vi "Main.vi"(8 "error in":errorcluster, 11 "CPU Percent in":refnum<class "Place Temperature.lvclass">) -> (0 "error out":errorcluster, 3 "CPU Percent out":refnum<class "Place Temperature.lvclass">)   [LabVIEW 2024, in "Place Temperature.lvclass"]
doc: "The <b>Queued Message Handler</b> of the Worker that owns this VI."
uses:
  Place Temperature.lvclass
  C:/Program Files (x86)/National Instruments/LabVIEW 2024/vi.lib/addons/_Workers/Library/Classes/Worker/Worker.lvclass
  rwr_Get Place Temperature Reply.ctl
  rqp_Set Place.ctl
  Place Temperature.lvclass/Place Temperature.ctl
  Controller/Controller.lvclass
  <vilib>/Python/Open Venv Python Session.vi
  <vilib>/addons/_Workers/Library/Classes/Worker/Worker.lvclass
  <vilib>/addons/_Workers/Library/Classes/Message Queue/Message Queue.lvclass
  Initialization Data.ctl
panel:
  out "Reply Data out":T1
  in  "Places":string(combo)="Baden, CH"
  in  "bGet Temperature":bool
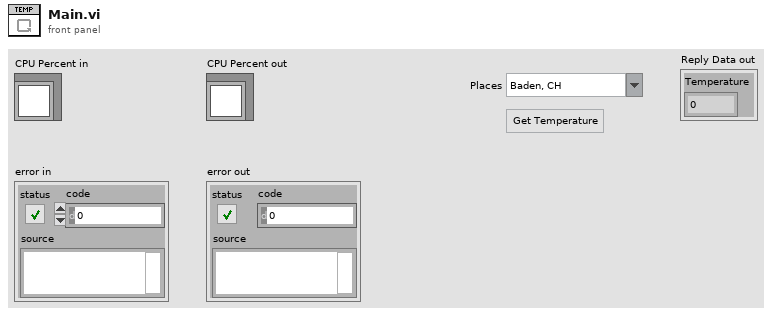
[diagram p1: front panel]
types:
  T1 = typedef "Place Temperature.lvclass/rwr_Get Place Temperature Reply.ctl" = cluster{"Temperature":dbl}
  T2 = typedef "Place Temperature.lvclass/Initialization Data.ctl" = cluster{"String":string, "Show Frontpanel":bool}
  T3 = enum32{"Invalid", "Standard", "Closed", "Hidden", "Minimized", "Maximized"}
  T4 = typedef "Place Temperature.lvclass/rqp_Set Place.ctl" = cluster{"Place":string}
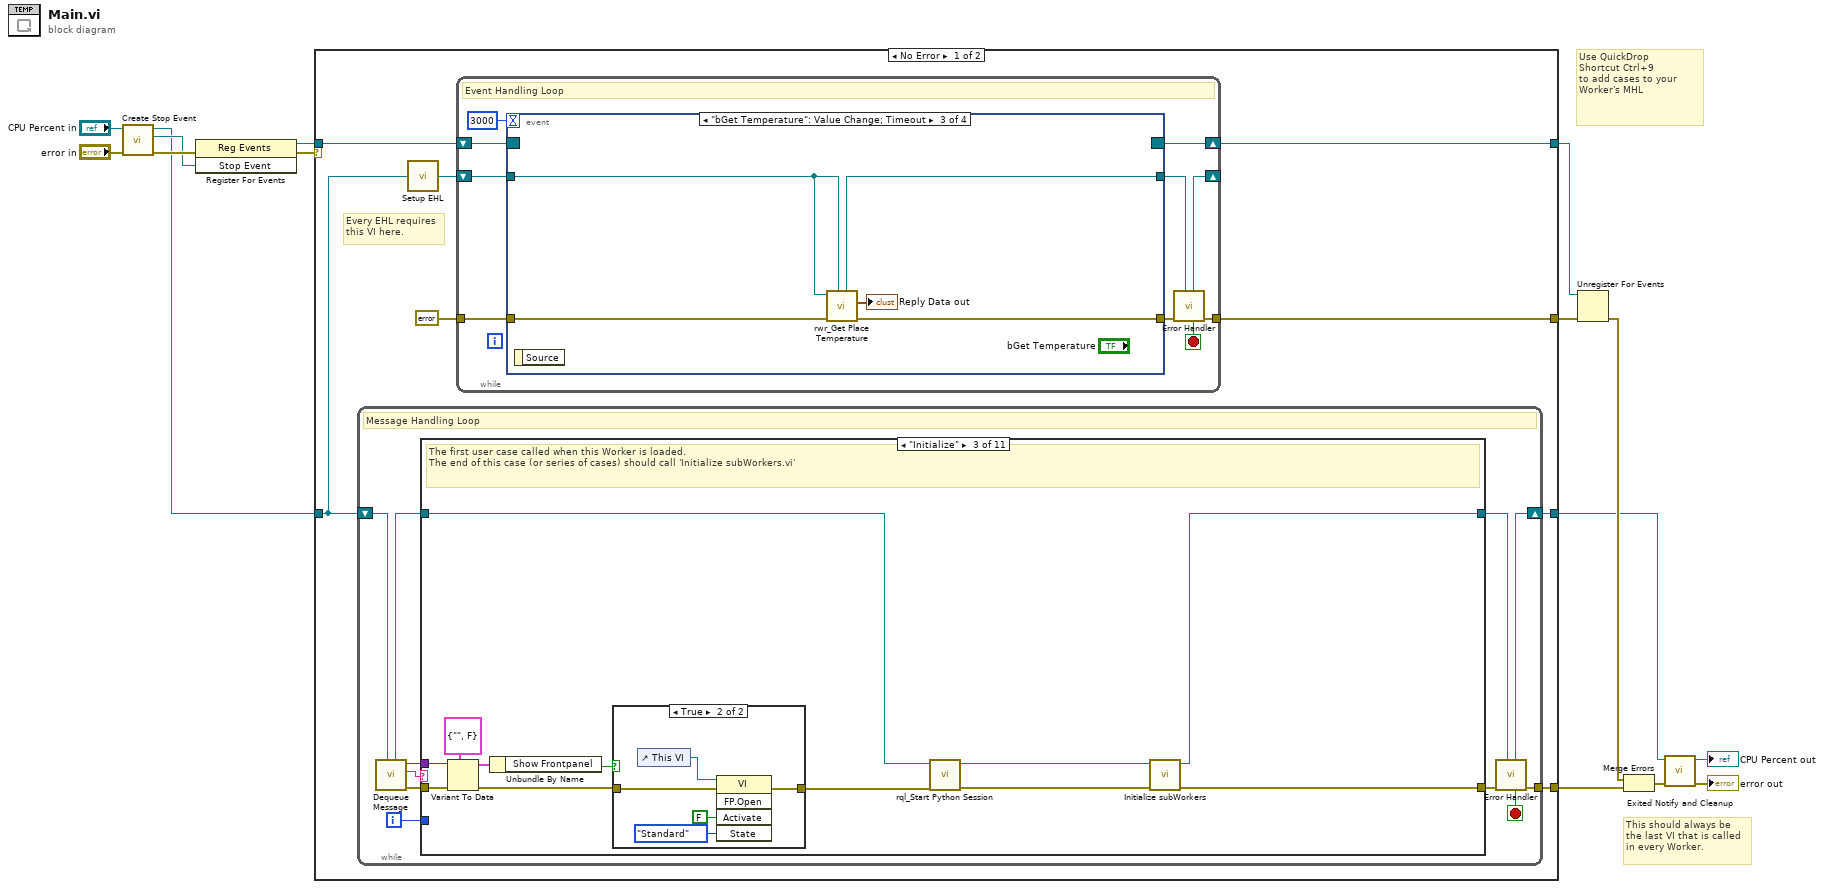
[diagram p0: block diagram]
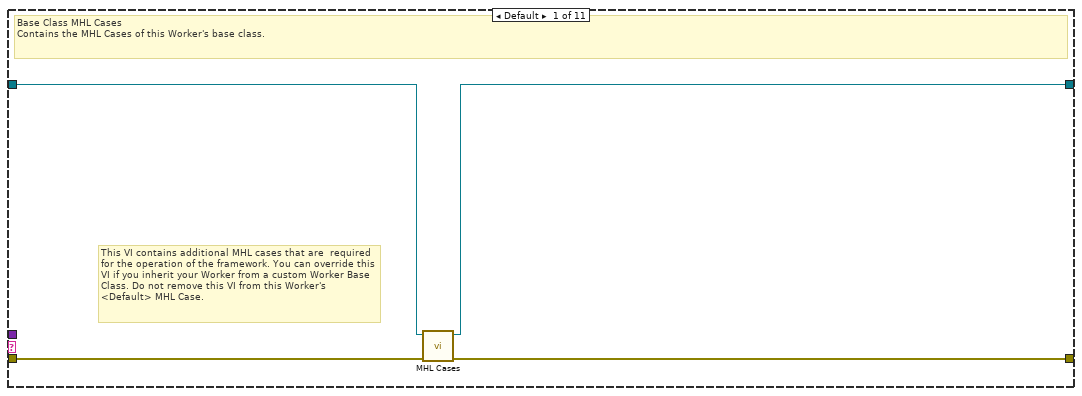
[diagram p2: hidden frame]
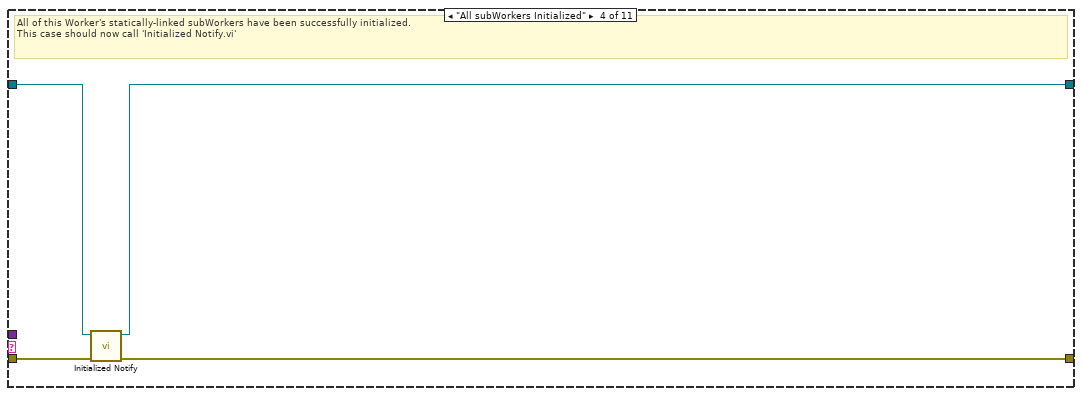
[diagram p5: hidden frame]
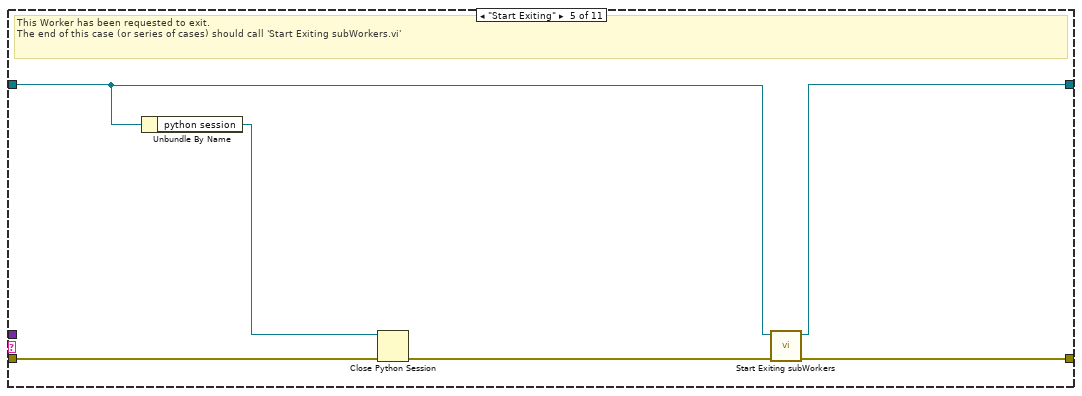
[diagram p6: hidden frame]
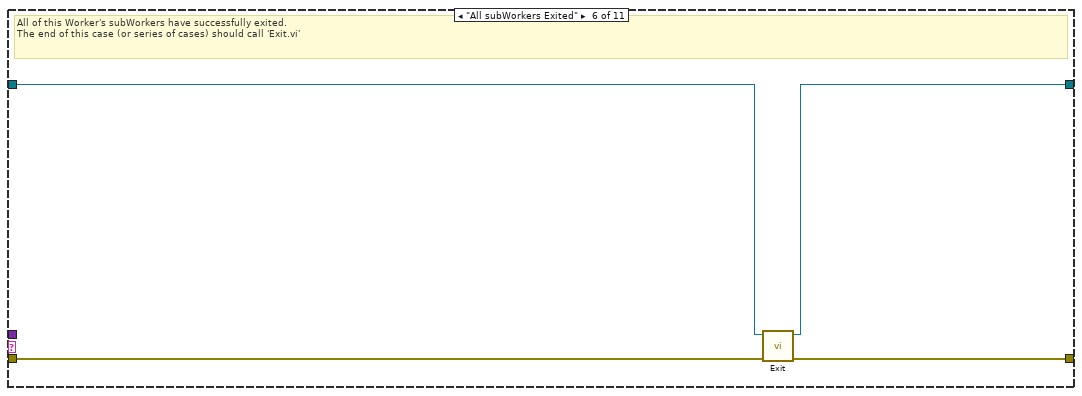
[diagram p7: hidden frame]
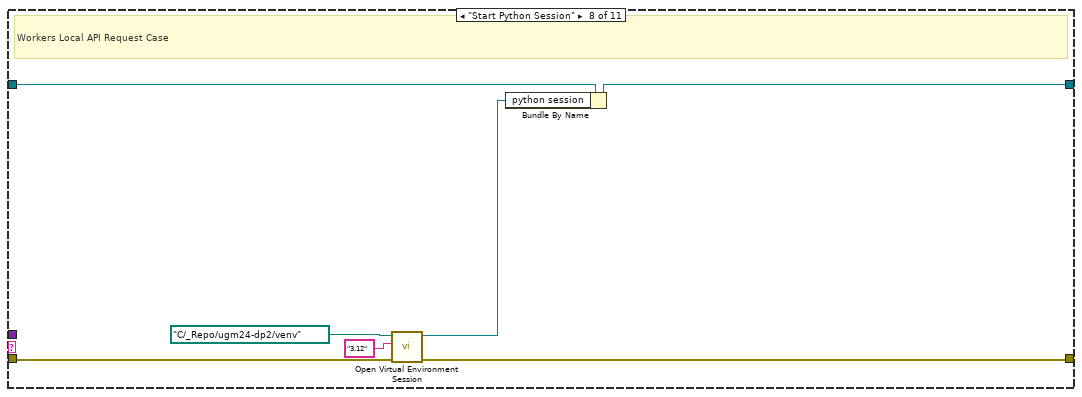
[diagram p9: hidden frame]
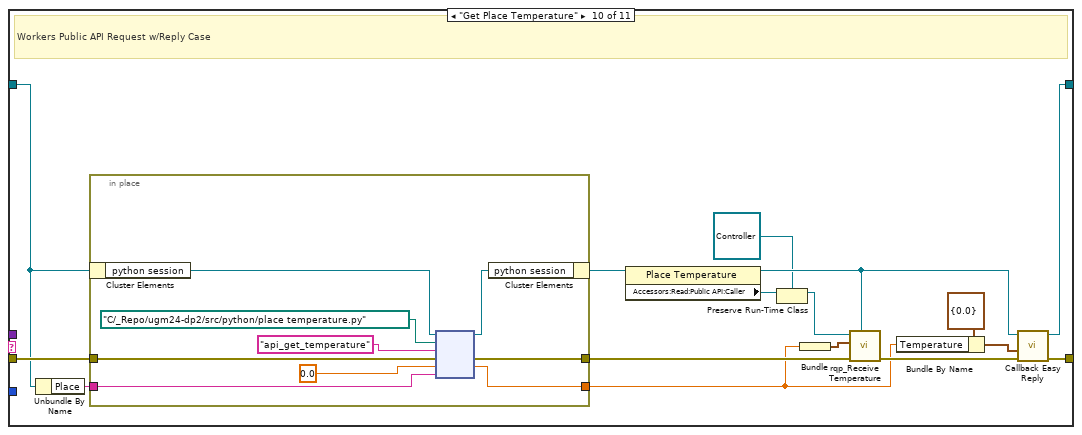
[diagram p11: hidden frame]
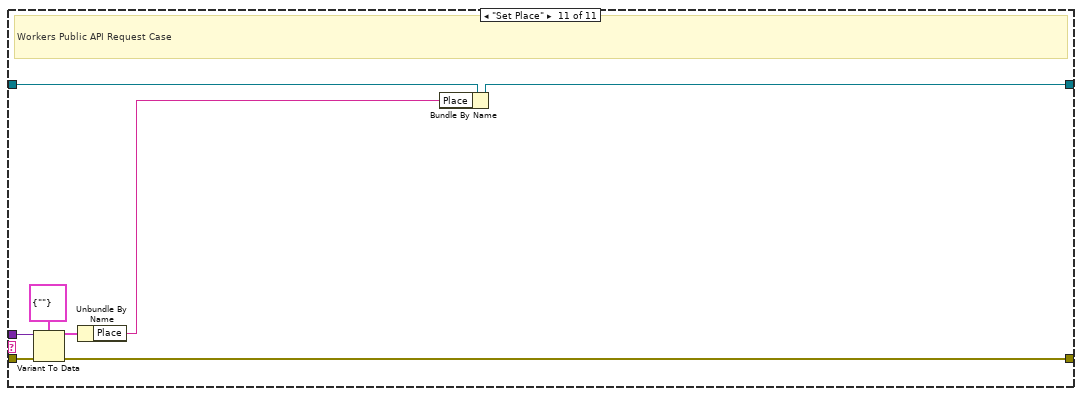
[diagram p12: hidden frame]
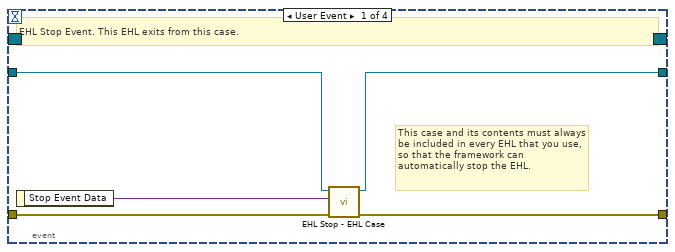
[diagram p13: hidden frame]
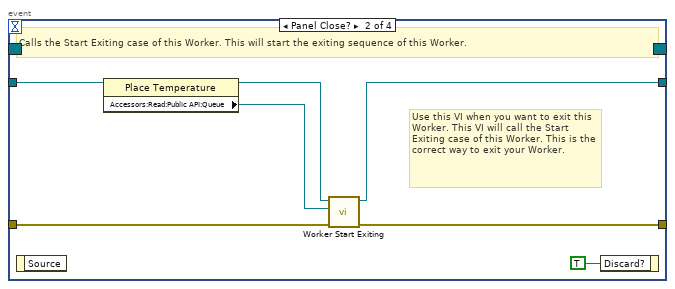
[diagram p14: hidden frame]
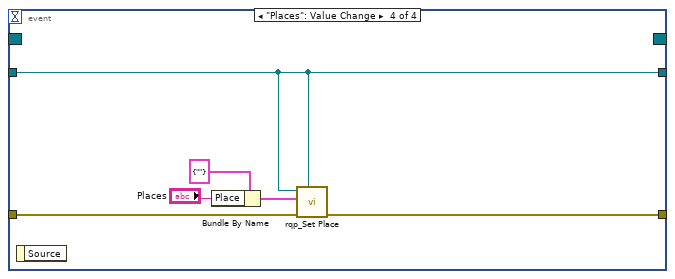
[diagram p15: hidden frame]
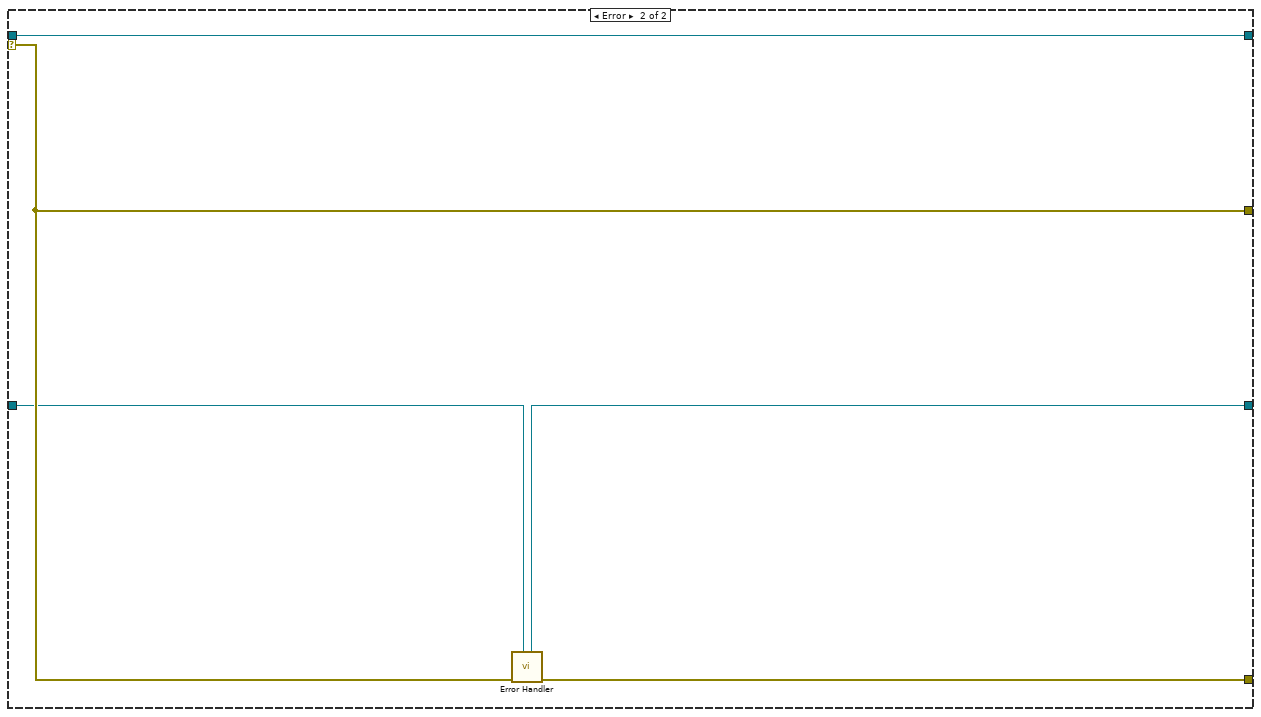
[diagram p16: hidden frame]
diagram:
  # "Use QuickDrop\nShortcut Ctrl+9\nto add cases to your\nWorker's MHL"
  # "This should always be the last VI that is called in every Worker."
  n1 = call-dynamic "Create Stop Event.vi"("error in"="error in", "Worker"="CPU Percent in") -> ("error out"=w10:errorcluster, "Stop Event"=w7:refnum<user-event>, "Worker out"=w4:refnum<class "Place Temperature.lvclass">)  [unwired: 7 in]
  n2 = register-events(error in=w10, w7) -> (reference out=w9:refnum<event-registration>, error out=w1:errorcluster)  [unwired: 1 in]
  n3 = case shown="No Error" w1 {
    tunnel: w4 -> [w18 w151]
    tunnel: [w16 w152] -> w8
    tunnel: w9 -> [w23 w153]
    tunnel: [w20 w154] -> w14
    tunnel: [w22 w153] -> w13
    tunnel: [w17 w150] -> w11
    selector: w1 -> [_ w154]
    frame No Error {
      # "Every EHL requires\nthis VI here."
      n4 = while {
        shift-right: [w32] -> w17
        shift-left: w18 -> [w34]
        tunnel: [w33] -> w16
        i -> [w25]
        stop <- w26 stop-if-true
        # "Message Handling Loop"
        n5 = call-dynamic "Dequeue Message.vi"("Worker"=w34) -> ("error out"=w31:errorcluster, "Case out"=w27:string, "Data out"=w24:variant, "Worker out"=w29:refnum<class "Place Temperature.lvclass">)  [unwired: 6 in, 1 out]
        n6 = case "Worker MHL Case Structure (DO NOT CHANGE LABEL NAME)" shown="\"Initialize\"" w27 {
          tunnel: w31 -> [w38 w39 w47 w60 w66 w72 w74 w78 w83 w96 w115]
          tunnel: [w37 w39 w52 w59 w68 w71 w74 w77 w83 w99 w114] -> w30
          tunnel: w29 -> [w36 w40 w48 w62 w65 w70 w73 w81 w82 w94 w116]
          tunnel: [w35 w40 w51 w61 w67 w69 w73 w76 w82 w98 w110] -> w28
          tunnel: w25 -> [_ _ _ _ _ _ _ _ _ _ _]
          tunnel: w24 -> [_ _ w46 _ _ _ _ _ _ _ w112]
          frame Default {
            # "This VI contains additional MHL cases that are  required for the operation of the framework. You can override this VI if you inherit your Worker from a custom Worker Base Class. Do not remove this VI from this Worker's <Default> MHL Case."
            # "Base Class MHL Cases\nContains the MHL Cases of this Worker's base class."
            n7 = call-dynamic "MHL Cases.vi"("error in"=w38, "Worker in"=w36) -> ("error out"=w37:errorcluster, "Worker out"=w35:refnum<class "Place Temperature.lvclass">)  [unwired: 8 in]
          }
          frame "------------ FRAMEWORK CASES -----------" {
            # "Start of Workers Framework Cases"
          }
          frame "Initialize" {
            # "The first user case called when this Worker is loaded.\nThe end of this case (or series of cases) should call 'Initialize subWorkers.vi'"
            n8 = Variant To Data(error in=w47, type=T2 {"String"="", "Show Frontpanel"=FALSE} ("Initialization Data"), Variant=w46) -> (data=w42:T2, error out=w44:errorcluster)
            n9 = Unbundle By Name(w42) -> ("Show Frontpanel"=w41:bool)
            n10 = case shown="True" w41 {
              tunnel: w44 -> [w53 w58]
              tunnel: [w53 w57] -> w43
              frame False {
              }
              frame True {
                n11 = control-ref of="This VI"() -> (w56:refnum<vi>)
                n12 = invoke class="VI" method="FP.Open"(reference=w56, error in=w58, "Activate"=FALSE ("Activate?"), "State"=T3."Standard") -> (error out=w57:errorcluster)  [unwired: 1 in, 4 out]
              }
            }
            n13 = call "rql_Start Python Session.vi"("error in"=w43, "CPU Percent in"=w48) -> ("error out"=w50:errorcluster, "dup CPU Percent out"=w49:refnum<class "Place Temperature.lvclass">)  [unwired: 8 in]
            n14 = call-dynamic "Initialize subWorkers.vi"("error in"=w50, "Worker"=w49) -> ("error out"=w52:errorcluster, "dup Worker out"=w51:refnum<class "Place Temperature.lvclass">)  [unwired: 8 in]
          }
          frame "All subWorkers Initialized" {
            # "All of this Worker's statically-linked subWorkers have been successfully initialized.\nThis case should now call 'Initialized Notify.vi'"
            n15 = call-dynamic "Initialized Notify.vi"("error in"=w60, "Worker"=w62) -> ("error out"=w59:errorcluster, "dup Worker out"=w61:refnum<class "Place Temperature.lvclass">)  [unwired: 8 in]
          }
          frame "Start Exiting" {
            # "This Worker has been requested to exit. \nThe end of this case (or series of cases) should call 'Start Exiting subWorkers.vi'"
            n16 = Unbundle By Name(w65) -> ("python session"=w63:refnum<k35>)
            n17 = Close Python Session(session in=w63, error in=w66) -> (11:w64:errorcluster)
            n18 = call-dynamic "Start Exiting subWorkers.vi"("error_in"=w64, "Worker"=w65) -> ("error out"=w68:errorcluster, "dup Worker out"=w67:refnum<class "Place Temperature.lvclass">)  [unwired: 8 in]
          }
          frame "All subWorkers Exited" {
            # "All of this Worker's subWorkers have successfully exited. \nThe end of this case (or series of cases) should call 'Exit.vi'"
            n19 = call-dynamic "Exit.vi"("error_in"=w72, "Worker"=w70) -> ("error out"=w71:errorcluster, "dup Worker out"=w69:refnum<class "Place Temperature.lvclass">)  [unwired: 8 in]
          }
          frame "------------- LOCAL API CASES -------------" {
            # "Start of Workers Local API Cases"
          }
          frame "Start Python Session" {
            # "Workers Local API Request Case"
            n20 = call-poly <vilib>:"Open Virtual Environment Session.vi"("error in (no error)"=w78, "Python version"="3.12", "Env path"=path "C:/_Repo/ugm24-dp2/venv") -> ("error out"=w77:errorcluster, "session out"=w75:refnum<k35>)  [unwired: 7 in]
            n21 = Bundle By Name(cluster=w81, "python session"=w75) -> (w76:refnum<class "Place Temperature.lvclass">)
          }
          frame "------------- PUBLIC API CASES -------------" {
            # "Start of Workers Public API Cases"
          }
          frame "Get Place Temperature" {
            # "Workers Public API Request w/Reply Case"
            n22 = Unbundle By Name(w94) -> ("Place"=w93:string)
            n23 = in-place {
              in-place-border: w96 -> [w108]
              in-place-border: [w102] -> w89
              in-place-border: [w101] -> w92
              in-place-border: w93 -> [w100]
              n24 = in-place-cluster #1(w94) -> ("python session"=w107:refnum<k35>)
              n25 = node(w107, path "C:/_Repo/ugm24-dp2/src/python/place temperature.py" ("module path"), "api_get_temperature" ("function name"), w108, 0.0, w100) -> (w103:refnum<k35>, w101:errorcluster, w102:dbl)  [unwired: 1 in, 2 out]
              n26 = in-place-cluster #1("python session"=w103) -> (w90:refnum<class "Place Temperature.lvclass">)
            }
            n27 = property class="Place Temperature"(reference=w90) -> (reference out=w87:refnum<class "Place Temperature.lvclass">, "Accessors:Read:Public API:Caller"=w86:refnum<class "Worker.lvclass">)  [unwired: 1 in, 1 out]
            n28 = Preserve Run-Time Class(object in=w86, 2:refnum<class "Controller.lvclass"> refnum ("Controller")) -> (object out=w84:refnum<class "Controller.lvclass">)  [unwired: 1 in, 1 out]
            n29 = Bundle(w89) -> (w88:cluster{dbl})  [unwired: 1 in]
            n30 = call "rqp_Receive Temperature.vi"("Caller in"=w87, "error in"=w92, "Data in"=w88, "Controller in"=w84) -> ("error out"=w91:errorcluster)  [unwired: 5 in, 2 out]
            n31 = Bundle By Name(cluster=T1 {"Temperature"=0.0} ("Reply Data"), "Temperature"=w89) -> (w95:T1)
            n32 = call-dynamic "Callback Easy Reply.vi"("error in"=w91, "Data"=w95, "Worker"=w87) -> ("error out"=w99:errorcluster, "dup Worker out"=w98:refnum<class "Place Temperature.lvclass">)  [unwired: 7 in]
          }
          frame "Set Place" {
            # "Workers Public API Request Case"
            n33 = Variant To Data(error in=w115, type=T4 {"Place"=""} ("Data"), Variant=w112) -> (data=w111:T4, error out=w114:errorcluster)
            n34 = Unbundle By Name(w111) -> ("Place"=w109:string)
            n35 = Bundle By Name(cluster=w116, "Place"=w109) -> (w110:refnum<class "Place Temperature.lvclass">)
          }
        }
        n36 = call-dynamic "Error Handler.vi"("Worker"=w28, "error_in"=w30) -> ("error out"=w33:errorcluster, "Stop Loop"=w26:bool, "Worker out"=w32:refnum<class "Place Temperature.lvclass">)  [unwired: 7 in]
      }
      n37 = call-dynamic "Setup EHL.vi"("Worker"=w18) -> ("Worker out"=w19:refnum<class "Place Temperature.lvclass">)  [unwired: 14 in]
      n38 = while "Event Handling Loop" {
        shift-right: [w126] -> w22
        shift-left: w23 -> [w125]
        tunnel: [w121] -> w20
        tunnel: errorcluster {"status"=FALSE, "code"=0, "source"=""} ("error constant") -> [w123]
        shift-right: [w119] -> _
        shift-left: w19 -> [w124]
        stop <- w118 stop-if-true
        # "Event Handling Loop"
        n39 = event shown="[2] \"bGet Temperature\": Value Change;  Timeout" {
          selector: w125 -> [_ _ _ _]
          dyn-events: [_ _ _ _] -> w126
          timeout: 3000 -> [_ _ _ _]
          tunnel: [w130 w137 w141 w149] -> w122
          tunnel: w123 -> [w131 w136 w142 w148]
          tunnel: w124 -> [w129 w135 w140 w144]
          tunnel: [w128 w134 w143 w144] -> w120
          event User Event {
            # "This case and its contents must always be included in every EHL that you use, so that the framework can automatically stop the EHL."
            # "EHL Stop Event. This EHL exits from this case."
            n40 = event-data() -> ("Stop Event Data"=w127:variant)  [unwired: 1 in]
            n41 = call-dynamic "EHL Stop - EHL Case.vi"("error in"=w131, "Stop Event Data"=w127, "Worker"=w129) -> ("error out"=w130:errorcluster, "Worker out"=w128:refnum<class "Place Temperature.lvclass">)  [unwired: 7 in]
          }
          event Panel Close? {
            # "Use this VI when you want to exit this Worker. This VI will call the Start Exiting case of this Worker. This is the correct way to exit your Worker."
            # "Calls the Start Exiting case of this Worker. This will start the exiting sequence of this Worker."
            n42 = event-data() -> ()  [unwired: 1 in, 1 out]
            n43 = property class="Place Temperature"(reference=w135) -> (reference out=w133:refnum<class "Place Temperature.lvclass">, "Accessors:Read:Public API:Queue"=w132:refnum<class "Message Queue.lvclass">)  [unwired: 1 in, 1 out]
            n44 = call-dynamic "Worker Start Exiting.vi"("error_in"=w136, "Message Queue"=w132, "Worker"=w133) -> ("error out"=w137:errorcluster, "dup Worker out"=w134:refnum<class "Place Temperature.lvclass">)  [unwired: 7 in]
            n45 = event-data("Discard?"=TRUE) -> ()  [unwired: 1 in, 1 out]
          }
          event "bGet Temperature": Value Change; Timeout {
            n46 = event-data() -> ()  [unwired: 1 in, 1 out]
            n47 = call "rwr_Get Place Temperature.vi"("Caller in"=w140, "error in"=w142, "Place Temperature in"=w140) -> ("error out"=w141:errorcluster, "Reply Data out"=→"Reply Data out":T1, "dup Caller out"=w143:refnum<class "Place Temperature.lvclass">)  [unwired: 5 in, 1 out]
          }
          event "Places": Value Change {
            n48 = event-data() -> ()  [unwired: 1 in, 1 out]
            n49 = Bundle By Name(cluster=T4 {"Place"=""} ("Data in"), "Place"="Places") -> (w146:T4)
            n50 = call "rqp_Set Place.vi"("Caller in"=w144, "error in"=w148, "Data in"=w146, "Place Temperature in"=w144) -> ("error out"=w149:errorcluster)  [unwired: 5 in, 2 out]
          }
        }
        n51 = call-dynamic "Error Handler.vi"("Worker"=w120, "error_in"=w122) -> ("error out"=w121:errorcluster, "Stop Loop"=w118:bool, "Worker out"=w119:refnum<class "Place Temperature.lvclass">)  [unwired: 7 in]
      }
    }
    frame Error {
      n52 = call-dynamic "Error Handler.vi"("Worker"=w151, "error_in"=w154) -> ("error out"=w152:errorcluster, "Worker out"=w150:refnum<class "Place Temperature.lvclass">)  [unwired: 7 in, 1 out]
    }
  }
  n53 = Unregister For Events(event registration refnum=w13, error in=w14) -> (error out=w15:errorcluster)
  n54 = Merge Errors(w15, w8) -> (w12:errorcluster)
  n55 = call-dynamic "Exited Notify and Cleanup.vi"("error_in"=w12, "Worker"=w11) -> ("error out"=→"error out":errorcluster, "dup Worker out"=→"CPU Percent out":refnum<class "Place Temperature.lvclass">)  [unwired: 8 in]
